vi "Calc_T_angle_Vel.vi"() -> ()   [LabVIEW 2010]
panel:
  out "Orders":dbl[](array[numeric])=[30.0, 79.0289488656166, 110.46550450061054, 134.59725313809946, 155.53515021929462] format="%.1f"
  out "Temperature orders Et1":dbl[](array[numeric])=[30.0, 75.0029581682178, 112.9090965112122, 140.82253230040124, 164.59369552853602] format="%.1f"
  out "dV to angle to":dbl=-2.1315141762734413e-07 format="%.1f"
  out "dV to 0 deg":dbl=-2.1315141762734413e-07 format="%.1f"
  out "T @  angle to":dbl=56.528812518598016 format="%.2g"
  out "d l @ angle to":dbl format="%_6g"
  in  "Angle to (deg)":dbl=5.0 format="%.3f"
  out "d l  @ max angle":dbl=-2.1315141762734413e-07 format="%_6g"
  out "d l  @ 0 deg":dbl=1.1354370466065689e-07 format="%_6g"
  out "T @ max angle":dbl=56.5121442947304 format="%.2g"
  in  "Et thickness":dbl=210.0 format="%.1f"
  in  "Wavelength":dbl=1.21 format="%_6g"
  out "Order":dbl=30.25551322702913 format="%.1f"
  out "Temperature vs refractive index":cluster{"Refr index raw":dbl[], "yi":dbl[]}[](graph)=[{"Refr index raw"=[3.51113, 3.51123, 3.51146, 3.51181, 3.51229, 3.51288, 3.51358, 3.51439, 3.51979, 3.52703, 3.53555, 3.54394], "yi"=[30.0, 40.0, 50.0, 60.0, 70.0, 80.0, 90.0, 100.0, 150.0, 200.0, 250.0, 295.0]}, {"Refr index raw"=[3.511673627651122], "yi"=[56.528812518598016]}]
  out "refr inx master from":dbl=3.511673627651122
  in  "Et T(K)":dbl=56.5
  out "dV to max angle":dbl=-2.1315141762734413e-07 format="%.1f"
  in  "Angle curr (deg)":dbl=5.0 format="%.3f"
  out "T @ 0 deg":dbl=56.53768737993274 format="%.2g"
  out "Out of  Range":bool
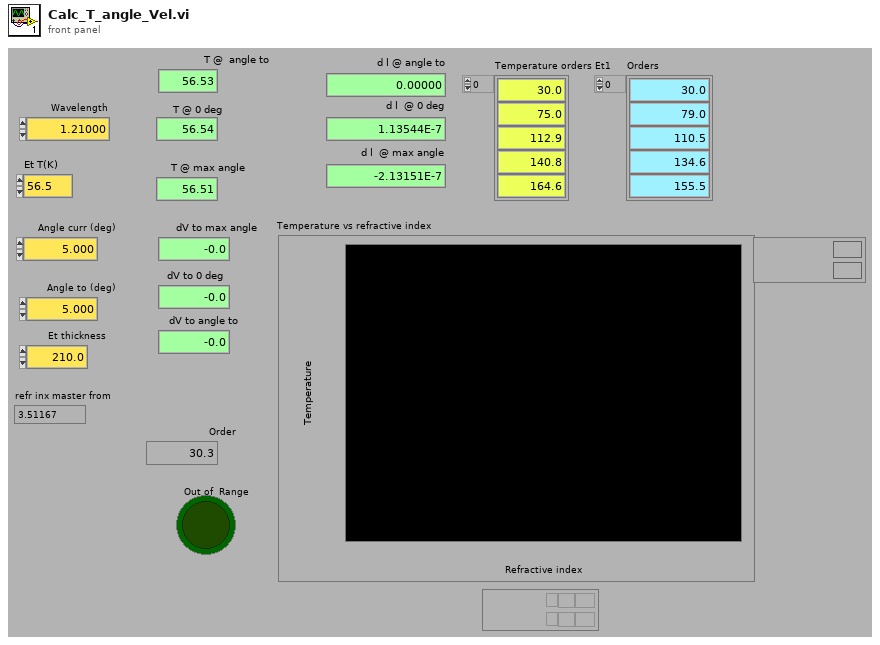
[diagram p1: front panel]
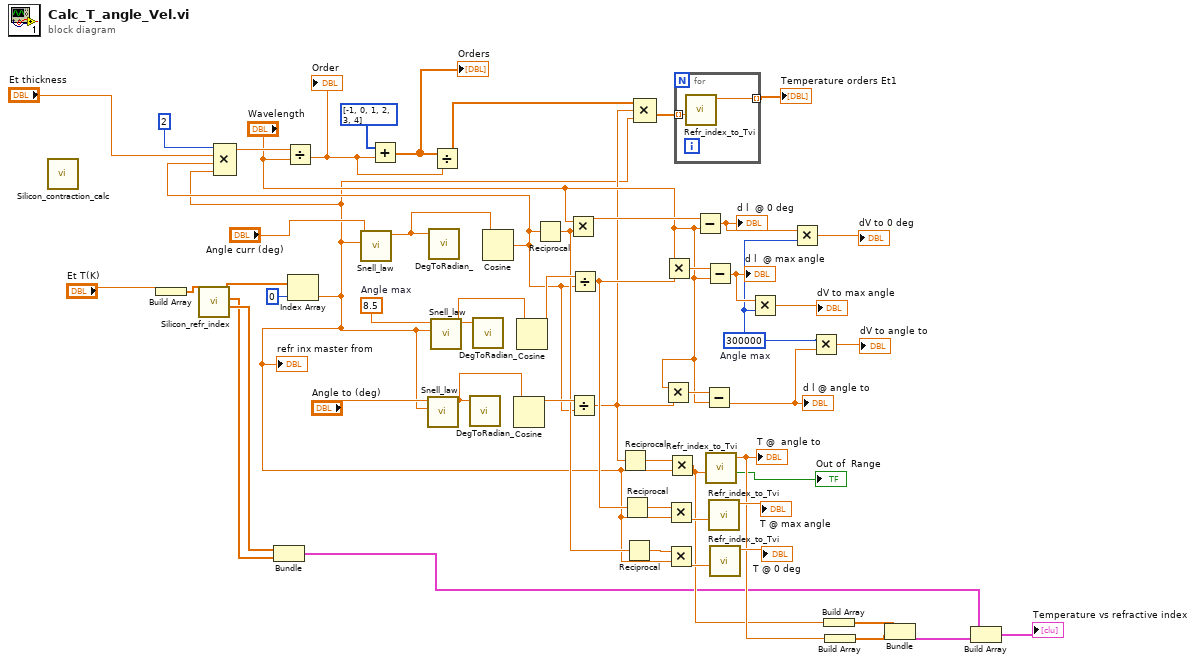
[diagram p0: block diagram]
diagram:
  w13 = 300000  # Angle max
  w41 = 8.5  # Angle max
  n1 = call "Silicon_contraction_calc.vi"() -> ()  [unwired: 6 in, 6 out]
  n2 = Build Array("Et T(K)") -> (w40:dbl[])
  n3 = call "Silicon_refr_index.vi"("Temperature"=w40) -> ("Refr index raw"=w53:dbl[], "T raw"=w52:dbl[], "Silicon refr index at T"=w48:dbl[])  [unwired: 8 in]
  n4 = Bundle("Refr index raw"=w53, "T raw"=w52) -> (w22:cluster{"Refr index raw":dbl[], "T raw":dbl[]})  [unwired: 1 in]
  n5 = Index Array(array=w48, index=0) -> (element=w6:dbl)
  "refr inx master from" <- w6
  n6 = call "Snell_law.vi"("Refr index"=w6, "Angle in ext (deg)"="Angle curr (deg)") -> ("Angle out int (rad)"=w21:dbl)  [unwired: 8 in, 1 out]
  n7 = call "Snell_law.vi"("Refr index"=w6, "Angle in ext (deg)"="Angle to (deg)") -> ("Angle out int (rad)"=w20:dbl)  [unwired: 8 in, 1 out]
  n8 = call "DegToRadian_.vi"("Angle deg"=w21) -> ()  [unwired: 4 in, 1 out]
  n9 = call "Snell_law.vi"("Refr index"=w6, "Angle in ext (deg)"=w41) -> ("Angle out int (rad)"=w19:dbl)  [unwired: 8 in, 1 out]
  n10 = call "DegToRadian_.vi"("Angle deg"=w20) -> ()  [unwired: 4 in, 1 out]
  n11 = call "DegToRadian_.vi"("Angle deg"=w19) -> ()  [unwired: 4 in, 1 out]
  n12 = Cosine(x=w21) -> (cos(x)=w8:dbl)
  n13 = Compound Arithmetic op=MULTIPLY(2 ("index"), "Et thickness", w8, w6) -> (w43:dbl)
  n14 = Divide(x=w43, y="Wavelength") -> (x/y=w45:dbl)
  "Order" <- w45
  n15 = Add(x=i32[] [-1, 0, 1, 2, 3, 4], y=w45) -> (x+y=w2:dbl[])
  "Orders" <- w2
  n16 = Divide(x=w2, y=w45) -> (x/y=w3:dbl[])
  n17 = Cosine(x=w20) -> (cos(x)=w32:dbl)
  n18 = Cosine(x=w19) -> (cos(x)=w38:dbl)
  n19 = Reciprocal(x=w8) -> (1/x=w30:dbl)
  n20 = Multiply(x="Wavelength", y=w30) -> (x*y=w37:dbl)
  n21 = Divide(x=w32, y=w8) -> (x/y=w7:dbl)
  n22 = Divide(x=w38, y=w8) -> (x/y=w31:dbl)
  n23 = Reciprocal(x=w7) -> (1/x=w11:dbl)
  n24 = Reciprocal(x=w31) -> (1/x=w10:dbl)
  n25 = Reciprocal(x=w30) -> (1/x=w9:dbl)
  n26 = Compound Arithmetic op=MULTIPLY(w3, w7, w6) -> (w5:dbl[])
  n27 = Multiply(x="Wavelength", y=w7) -> (x*y=w34:dbl)
  n28 = Multiply(x="Wavelength", y=w31) -> (x*y=w36:dbl)
  n29 = Multiply(x=w10, y=w6) -> (x*y=w28:dbl)
  n30 = Multiply(x=w9, y=w6) -> (x*y=w29:dbl)
  n31 = Multiply(x=w11, y=w6) -> (x*y=w24:dbl)
  n32 = for {
    tunnel: w5 -> [w56] mode=indexing
    tunnel: [w55] -> w4 mode=indexing
    n33 = call "Refr_index_to_Tvi.vi"("refr inx"=w56) -> ("T tune to"=w55:dbl)  [unwired: 9 in, 1 out]
  }
  "Temperature orders Et1" <- w4
  n34 = Subtract(x=w37, y="Wavelength") -> (x-y=w16:dbl)
  "d l  @ 0 deg" <- w16
  n35 = Subtract(x=w34, y="Wavelength") -> (x-y=w14:dbl)
  "d l @ angle to" <- w14
  n36 = Subtract(x=w36, y="Wavelength") -> (x-y=w18:dbl)
  "d l  @ max angle" <- w18
  n37 = call "Refr_index_to_Tvi.vi"("refr inx"=w24) -> ("Out of  Range"=→"Out of  Range":bool, "T tune to"=w25:dbl)  [unwired: 9 in]
  "T @  angle to" <- w25
  n38 = call "Refr_index_to_Tvi.vi"("refr inx"=w28) -> ("T tune to"=→"T @ max angle":dbl)  [unwired: 9 in, 1 out]
  n39 = call "Refr_index_to_Tvi.vi"("refr inx"=w29) -> ("T tune to"=→"T @ 0 deg":dbl)  [unwired: 9 in, 1 out]
  n40 = Multiply(x=w18, y=w13) -> (x*y=→"dV to max angle":dbl)
  n41 = Multiply(x=w16, y=w13) -> (x*y=→"dV to 0 deg":dbl)
  n42 = Multiply(x=w13, y=w14) -> (x*y=→"dV to angle to":dbl)
  n43 = Build Array(w24) -> (w50:dbl[])
  n44 = Build Array(w25) -> (w51:dbl[])
  n45 = Bundle(w50, w51) -> (w54:cluster{dbl[], dbl[]})  [unwired: 1 in]
  n46 = Build Array(w22, w54) -> (→"Temperature vs refractive index":cluster{"Refr index raw":dbl[], "T raw":dbl[]}[])
